vi "XML_read_cluster.vi"(0 "Name":string="lowerBound", 1 "XML":string="       <member>\n            <name>lowerBound</name>\n           <value><i4>18</i4></value>\n       </member>\n        <member>\n           <name>upperBound</name>\n           <value><i4>139</i4></value>\n         </member>\n\n") -> (2 "ParsingErrors":string, 3 "Value":variant=variant(i32 18), 4 "Type":T1(ring))   [LabVIEW 2010]
panel:
  out "found?":bool=TRUE
  out "Rest":string="\n        <member>\n           <name>upperBound</name>\n           <value><i4>139</i4></value>\n         </member>\n\n"
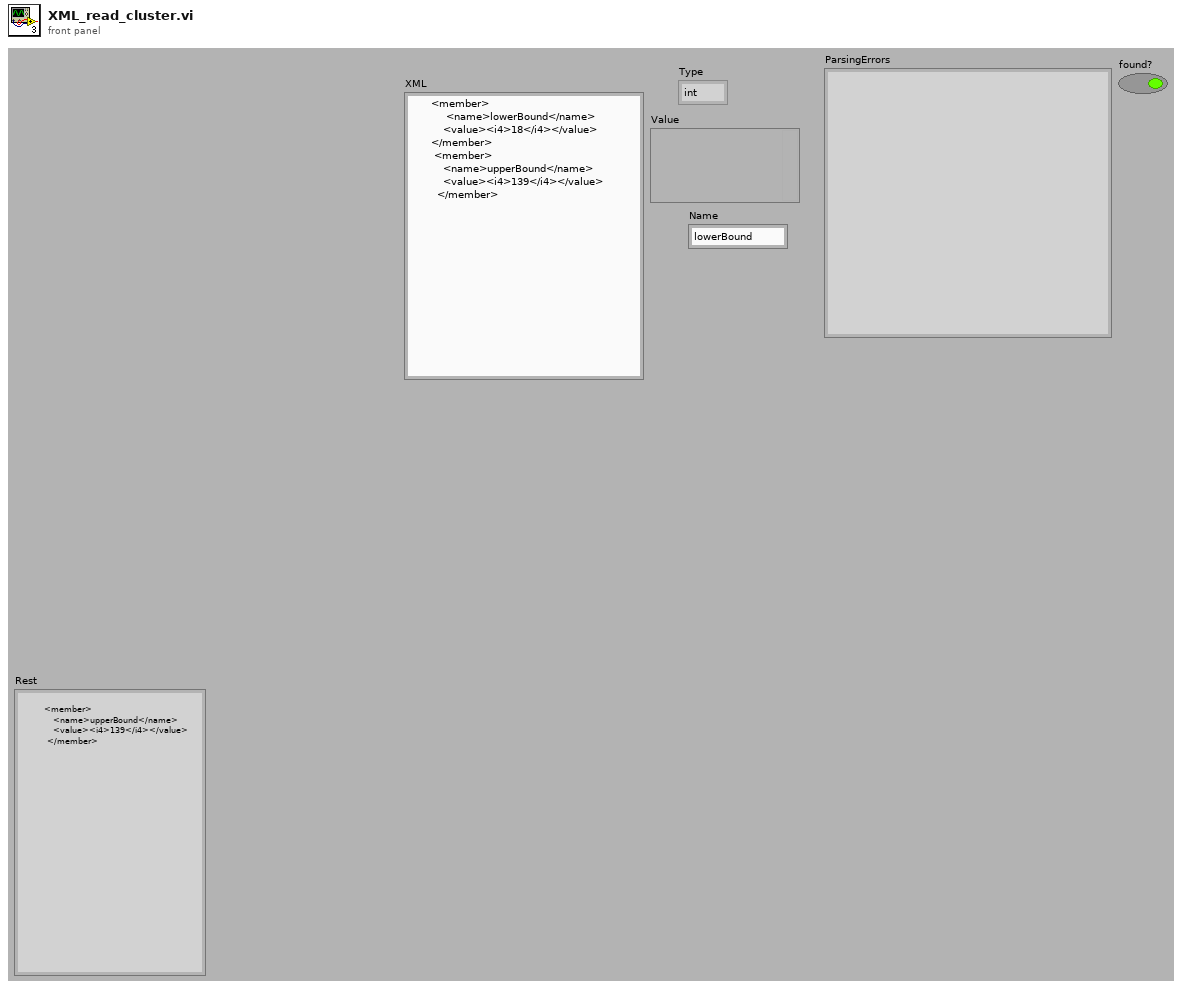
[diagram p1: front panel]
types:
  T1 = enum16{"int", "boolean", "string", "double", "dateTime", "base64", "struct", "array"}
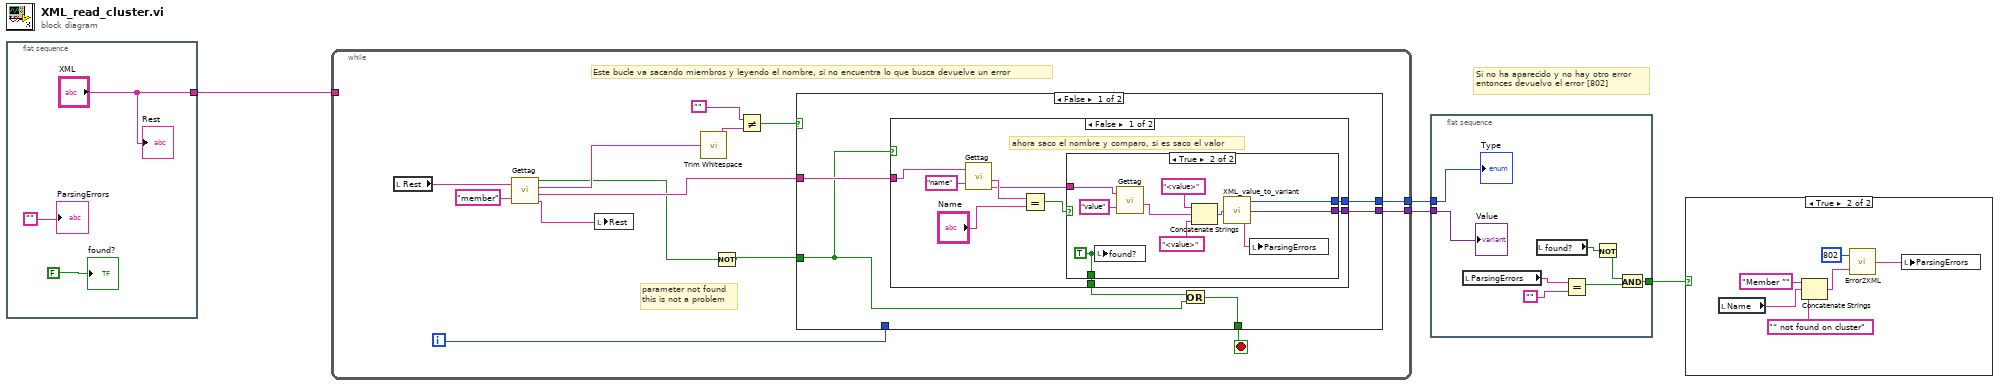
[diagram p0: block diagram]
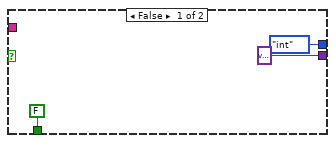
[diagram p3: hidden frame]
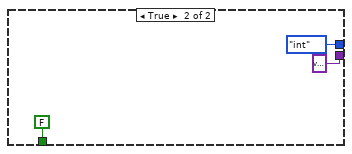
[diagram p4: hidden frame]
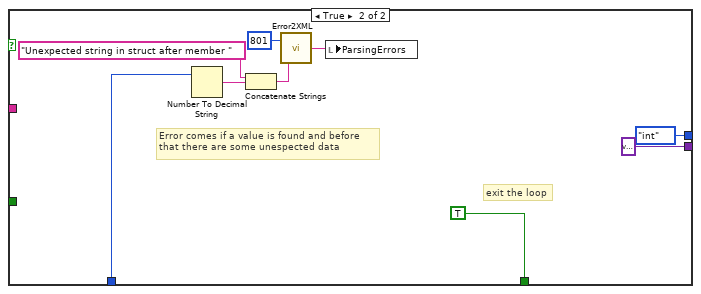
[diagram p5: hidden frame]
diagram:
  # "Si no ha aparecido y no hay otro error \nentonces devuelvo el error [802]"
  n1 = flat-sequence {
    tunnel: ["XML"] -> w4
    frame #0 {
      "ParsingErrors" <- ""
      "Rest" <- "XML"
      "found?" <- FALSE
    }
  }
  n2 = while {
    tunnel: w4 -> [_]
    tunnel: [w9] -> w3
    tunnel: [w8] -> w2
    i -> [w18]
    stop <- w17 stop-if-true
    # "Este bucle va sacando miembros y leyendo el nombre, si no encuentra lo que busca devuelve un error"
    # "parameter not found\nthis is not a problem"
    n3 = local read "Rest"() -> (w15:string)
    n4 = call "Gettag.vi"("TagName"="member", "XML"=w15) -> ("AfterTag"=w13:string, "InsideTag"=w14:string, "BeforeTag"=w12:string, "Found?"=w10:bool)
    n5 = local write "Rest"(w13) -> ()
    n6 = call <vilib>:"Trim Whitespace.vi"("string"=w12) -> ("trimmed string"=w20:string)  [unwired: 1 in]
    n7 = Not(x=w10) -> (.not. x?=w11:bool)
    n8 = Not Equal?(x="", y=w20) -> (x != y?=w19:bool)
    n9 = case shown="False" w19 {
      tunnel: w18 -> [_ w60]
      tunnel: w11 -> [w24 _]
      tunnel: w14 -> [w27 _]
      tunnel: [w23 TRUE] -> w17
      tunnel: [w26 T1."int" ("Type")] -> w9
      tunnel: [w25 variant ("Value")] -> w8
      frame False {
        n10 = case shown="False" w24 {
          tunnel: w27 -> [w36 _]
          tunnel: [w30 T1."int" ("Type")] -> w26
          tunnel: [w29 variant ("Value")] -> w25
          tunnel: [w28 FALSE ("found?")] -> w22
          frame False {
            # "ahora saco el nombre y comparo, si es saco el valor"
            n11 = call "Gettag.vi"("TagName"="name", "XML"=w36) -> ("AfterTag"=w31:string, "InsideTag"=w34:string)  [unwired: 2 out]
            n12 = Equal?(x=w34, y="Name") -> (x = y?=w32:bool)
            n13 = case shown="True" w32 {
              tunnel: w31 -> [_ w49]
              tunnel: [T1."int" ("Type") w43] -> w30
              tunnel: [variant ("Value") w42] -> w29
              tunnel: [FALSE ("found?") w40] -> w28
              frame False {
              }
              frame True {
                w40 = TRUE ("found?")
                n14 = local write "found?"(w40) -> ()
                n15 = call "Gettag.vi"("TagName"="value", "XML"=w49) -> ("InsideTag"=w44:string)  [unwired: 3 out]
                n16 = Concatenate Strings("<value>" ("string"), w44, "<value>" ("string")) -> (w47:string)
                n17 = call "XML_value_to_variant.vi"("XML-param"=w47) -> ("ParsingErrors"=w41:string, "Value"=w42:variant, "Type"=w43:T1)
                n18 = local write "ParsingErrors"(w41) -> ()
              }
            }
          }
          frame True {
          }
        }
        n19 = Or(x=w22, y=w24) -> (x .or. y?=w23:bool)
      }
      frame True {
        # "Error comes if a value is found and before\nthat there are some unespected data"
        # "exit the loop"
        n20 = Number To Decimal String(number=w60) -> (decimal integer string=w59:string)  [unwired: 1 in]
        n21 = Concatenate Strings("Unexpected string in struct after member " ("FailDescriptor"), w59) -> (w56:string)
        n22 = call "Error2XML.vi"("FailDescriptor"=w56, "FailID"=801) -> ("ErrorXML"=w53:string)
        n23 = local write "ParsingErrors"(w53) -> ()
      }
    }
  }
  n24 = flat-sequence {
    tunnel: w3 -> [w69]
    tunnel: w2 -> [w68]
    tunnel: [w62] -> w1
    frame #0 {
      n25 = local read "ParsingErrors"() -> (w67:string)
      n26 = local read "found?"() -> (w64:bool)
      n27 = Equal?(x=w67, y="") -> (x = y?=w65:bool)
      n28 = Not(x=w64) -> (.not. x?=w63:bool)
      n29 = And(x=w63, y=w65) -> (x .and. y?=w62:bool)
      "Type" <- w69
      "Value" <- w68
    }
  }
  n30 = case shown="True" w1 {
    frame False {
    }
    frame True {
      n31 = local read "Name"() -> (w71:string)
      n32 = Concatenate Strings("Member ”" ("string"), w71, "“ not found on cluster" ("string")) -> (w73:string)
      n33 = call "Error2XML.vi"("FailDescriptor"=w73, "FailID"=802) -> ("ErrorXML"=w74:string)
      n34 = local write "ParsingErrors"(w74) -> ()
    }
  }
